vi "GHV232 CRAB.vi"() -> ()   [LabVIEW 2017]
doc: "The Basic Serial Read and Write example performs a Serial Port Read, a Serial Port Write, or a combination of these actions. The user selects the actions (read or write) on the front panel. If both are selected, the VI will write the data first, read data, and then close the VISA session that is opened to the port. This VI will wait until the specified number of bytes is received at the port. Only the number of bytes specified will be read.\n\nINSTRUCTIONS:\n1) Select the serial resource and configuration parameters (baud rate, data bits, parity, stop bits, flow control).\n2) Select the operations to be performed. \n3) Connect the serial port to your device. If no device is available, perform a loopback test by doing one of the following. Short pins 2 and 3 on a RS-232 cable or short pin 4 to pin 8 and pin 5 to pin 9 on a RS-485/422 cable. \n4) Run the VI to see the data read. (The \"read string\" will match the \"string to write\" if a loopback test was performed.)\n\nNote: The parameters set for the serial port must match the parameters of the connected instrument or device. In this example, the bytes to read parameter specifies the number of bytes that the serial port reads. If there were more bytes at the port than the number specified in bytes to read, those bytes would not be read. Also, if you specify to read more bytes than the number of bytes actually read, you might receive a timeout error message.\n\nOn the block diagram, the Configure Serial Port VI sets the configuration parameters. The front panel displays the controls used to configure the basic parameters, such as baud rate, data bits, and parity. Constants configure the other parameters the user probably does not need set. After the VISA Configure Serial Port VI opens the VISA session and configures the port, the VI passes the VISA resource name to other VIs that perform operations on that VISA resource. The VISA Write function sends a command to the serial device and the VISA Read function returns data based on the command. The VISA Close function then closes the reference to the serial device. It is important to close the reference; otherwise communication through with that port through protocols other than VISA might not be possible."
uses:
  <vilib>/Instr/_visa.llb/VISA Configure Serial Port (Instr).vi
  <vilib>/Analysis/1siggen.llb/Ramp Pattern by Delta.vi
  <vilib>/Analysis/NI_AALBase.lvlib
panel:
  in  "Send 3":bool
  out "Message 3":string
  in  "Reset 3":bool
  out "HV On 3":bool
  out "Fault 3":bool
  out "Vmode 3":bool
  out "Imode 3":bool
  out "Voltage Monitor 3":dbl format="%#.2g"
  out "Current Monitor 3":dbl format="%#.2g"
  in  "High Voltage 3":bool
  in  "Voltage Progra3":dbl min=0.0 max=100.0 step=0.1 format="%#.2g"
  in  "Current Progra3":dbl min=0.0 max=100.0 step=0.1 format="%#.2g"
  in  "Version 3":bool
  in  "?":bool
  in  "Baud Rate 3":u16=9600 min=1200 max=19200 step=1200
  in  "Flow Control 3":u16(ring) items=["None"=0, "XON/XOFF"=1, "RTS/CTS"=2, "DTR/DSR"=4]
  in  "Stop Bits 3":u16(ring)=10 items=["1.0"=10, "1.5"=15, "2.0"=20]
  in  "Parity 3":u16(ring) items=["None", "Odd", "Even", "Mark", "Space"]
  in  "Data Bits 3":u16=8 min=5 max=8 step=1
  in  "VISA resource name 3":refnum<visa-resource-name>="COM1"
  in  "Send 2":bool
  out "Message 2":string
  in  "Reset 2":bool
  out "HV On 2":bool
  out "Fault 2":bool
  out "Vmode 2":bool
  out "Imode 2":bool
  out "Voltage Monitor 2":dbl format="%#.2g"
  out "Current Monitor 2":dbl format="%#.2g"
  in  "High Voltage 2":bool
  in  "Voltage Program 2":dbl min=0.0 max=100.0 step=0.1 format="%#.2g"
  in  "Current Program 2":dbl min=0.0 max=100.0 step=0.1 format="%#.2g"
  in  "Version 2":bool
  in  "?":bool
  in  "Baud Rate 2":u16=9600 min=1200 max=19200 step=1200
  in  "Flow Control 2":u16(ring) items=["None"=0, "XON/XOFF"=1, "RTS/CTS"=2, "DTR/DSR"=4]
  in  "Stop Bits 2":u16(ring)=10 items=["1.0"=10, "1.5"=15, "2.0"=20]
  in  "Parity 2":u16(ring) items=["None", "Odd", "Even", "Mark", "Space"]
  in  "Data Bits 2":u16=8 min=5 max=8 step=1
  in  "VISA resource name 2":refnum<visa-resource-name>="COM1"
  in  "?":bool
  in  "Version":bool
  in  "Baud Rate":u16=9600 min=1200 max=19200 step=1200
  in  "Reset":bool
  in  "Send":bool
  in  "Flow Control":u16(ring) items=["None"=0, "XON/XOFF"=1, "RTS/CTS"=2, "DTR/DSR"=4]
  in  "Stop Bits":u16(ring)=10 items=["1.0"=10, "1.5"=15, "2.0"=20]
  in  "Parity":u16(ring) items=["None", "Odd", "Even", "Mark", "Space"]
  in  "Data Bits":u16=8 min=5 max=8 step=1
  in  "High Voltage":bool
  in  "Voltage Program":dbl min=0.0 max=100.0 step=0.1 format="%#.2g"
  in  "Current Program":dbl min=0.0 max=100.0 step=0.1 format="%#.2g"
  in  "VISA resource name":refnum<visa-resource-name>="COM1"
  out "Message":string
  out "Fault":bool
  out "HV On":bool
  out "Imode":bool
  out "Vmode":bool
  out "Current Monitor":dbl format="%#.2g"
  out "Voltage Monitor":dbl format="%#.2g"
  # "GHV232 Example:  When this example is run, it will continuously query the power supply and update the the digital and\nanalog monitors (0-100%).  The Send Program button will send the the programs (0-100%) and the high voltage enable\nsignal to the power supply.  A Power Supply Reset will set both voltage and current programs to zero and turn the high \nvoltage off.  The power supply will respond with 'Acknowledge OK' for both a Send Program and Power Supply Reset.  A \nFirmware Version Request will display the current revision of the Power Supply Firmware.  Disconnect will close the serial \nport and stop execution.  HV On, Fault, V/I Mode LEDs may not be available on all Power Supplies."
  # "GHV PowerSupply 6 EL+"
  # "GHV PowerSupply 5 FIELDCAGE"
  # "GHV PowerSupply 4 EL++"
  # "Programs"
  # "Programs"
  # "Programs"
  # "Configuration"
  # "Configuration"
  # "Configuration"
  # "%"
  # "On"
  # "On"
  # "On"
  # "%"
  # "%"
  # "%"
  # "Off"
  # "Off"
  # "Off"
  # "%"
  # "%"
  # "%"
  # "Monitors"
  # "Monitors"
  # "Monitors"
  # "%"
  # "%"
  # "%"
  # "%"
  # "%"
  # "%"
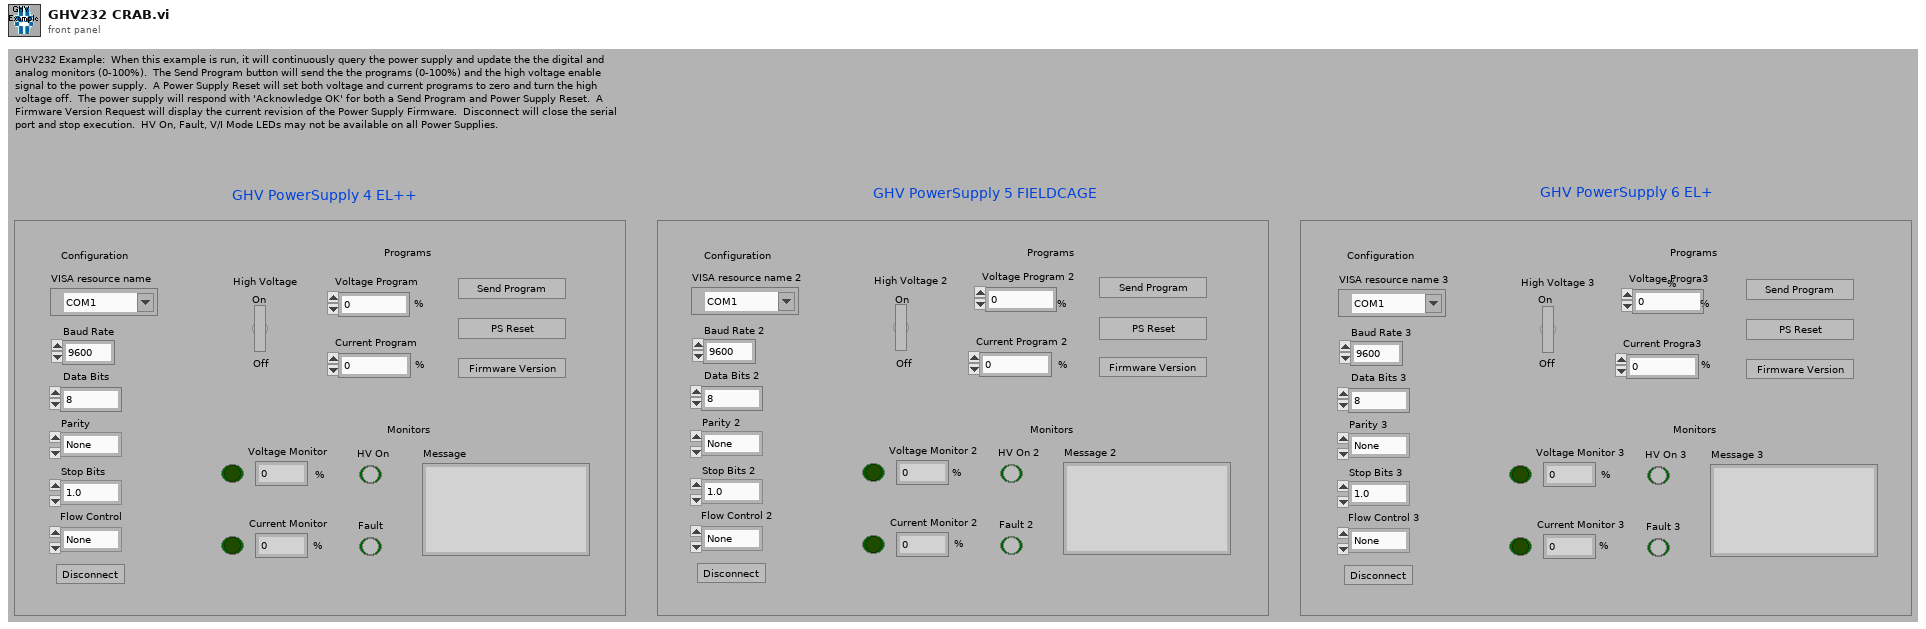
[diagram p1: front panel]
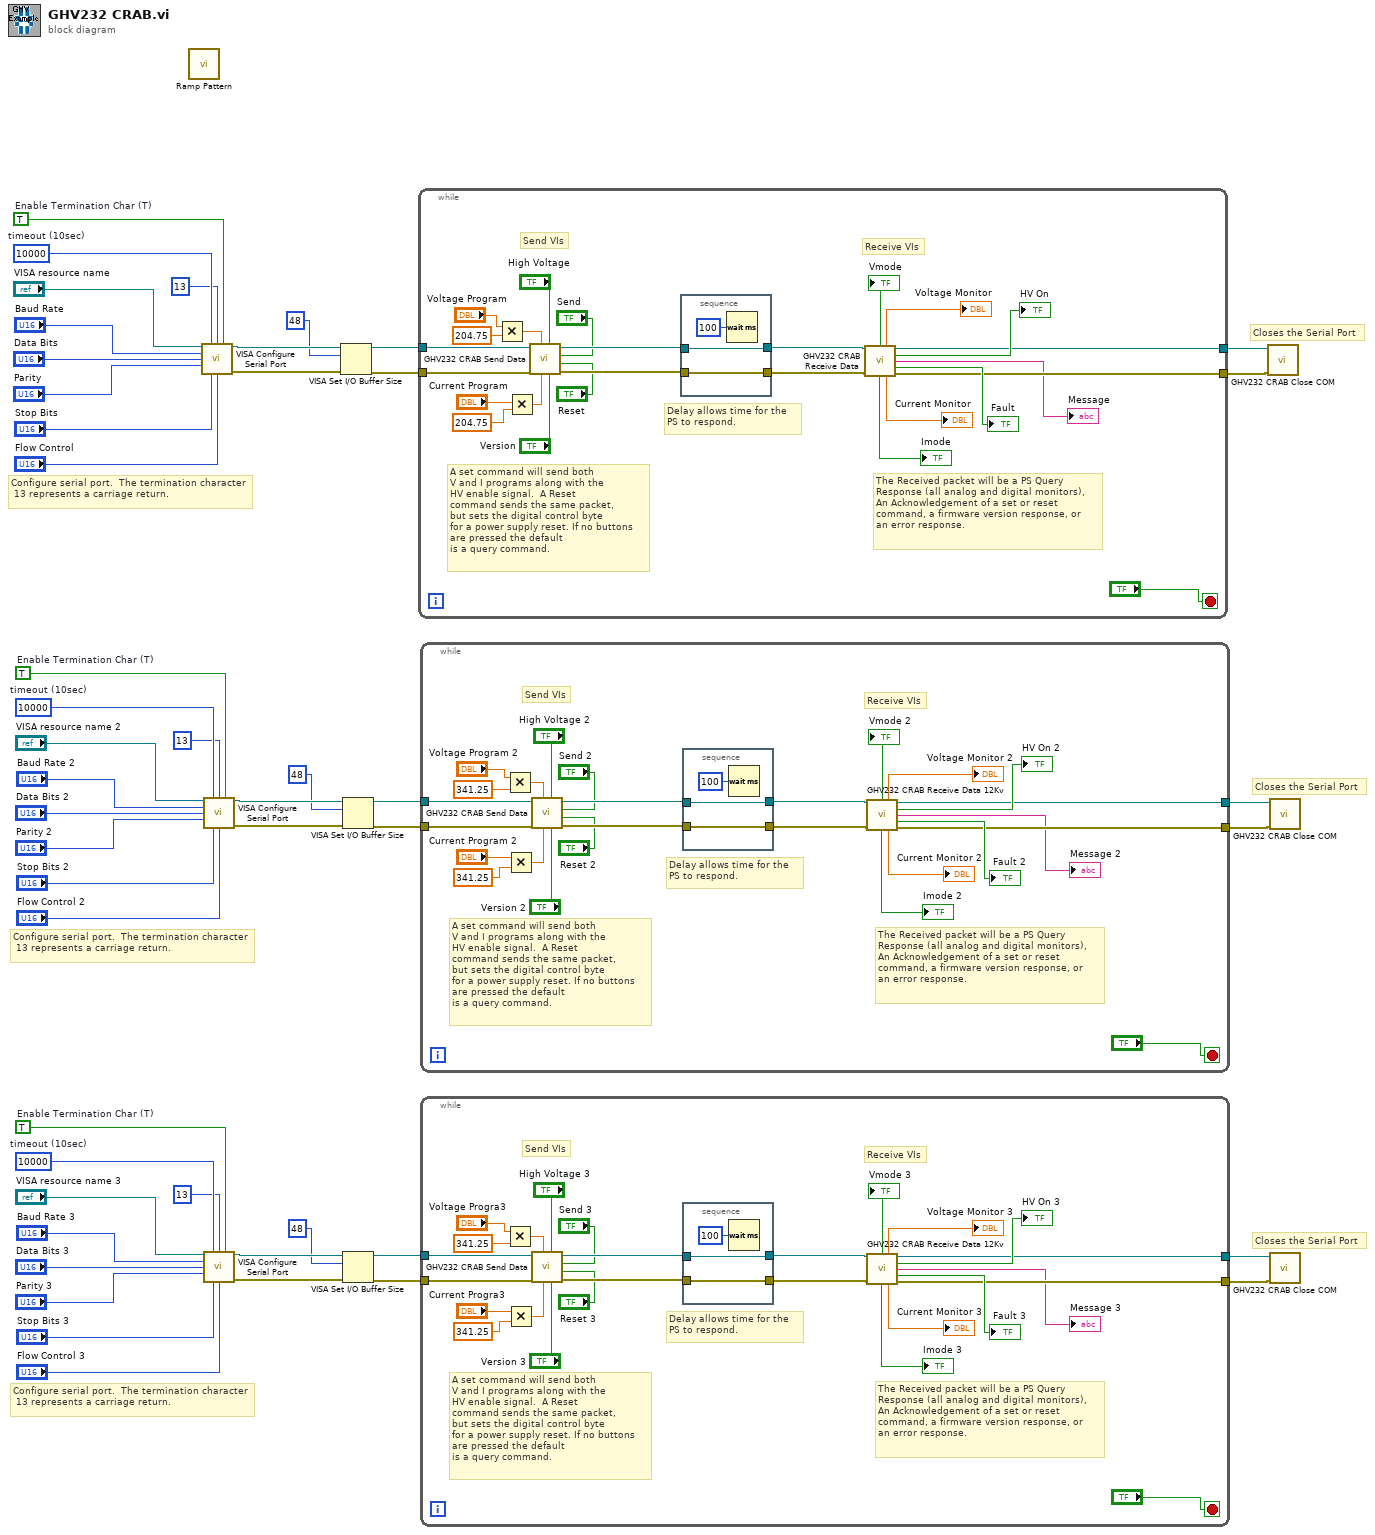
[diagram p0: block diagram]
diagram:
  w13 = TRUE  # Enable Termination Char (T)
  w14 = u32 10000  # timeout (10sec)
  w29 = TRUE  # Enable Termination Char (T)
  w30 = u32 10000  # timeout (10sec)
  w45 = TRUE  # Enable Termination Char (T)
  w46 = u32 10000  # timeout (10sec)
  # "Closes the Serial Port"
  # "Configure serial port.  The termination character\n 13 represents a carriage return."
  # "Closes the Serial Port"
  # "Configure serial port.  The termination character\n 13 represents a carriage return."
  # "Closes the Serial Port"
  # "Configure serial port.  The termination character\n 13 represents a carriage return."
  n1 = call-poly <vilib>:"Ramp Pattern.vi"() -> ()  [unwired: 9 in, 3 out]
  n2 = call-poly "VISA Configure Serial Port"("VISA resource name"="VISA resource name", "timeout (10sec)"=w46, "termination char\n(0xA = '\\n' = LF)"=13, "Enable Termination\nChar (T)"=w45, "baud rate (9600)"="Baud Rate", "data bits (8)"="Data Bits", "parity (0:none)"="Parity", "stop bits (10: 1 bit)"="Stop Bits", "flow control (0:none)"="Flow Control") -> ("VISA resource name out"=w35:refnum<visa-resource-name>, "error out"=w34:errorcluster)  [unwired: 5 in]
  n3 = call-poly "VISA Configure Serial Port"("VISA resource name"="VISA resource name 2", "timeout (10sec)"=w30, "termination char\n(0xA = '\\n' = LF)"=13, "Enable Termination\nChar (T)"=w29, "baud rate (9600)"="Baud Rate 2", "data bits (8)"="Data Bits 2", "parity (0:none)"="Parity 2", "stop bits (10: 1 bit)"="Stop Bits 2", "flow control (0:none)"="Flow Control 2") -> ("VISA resource name out"=w19:refnum<visa-resource-name>, "error out"=w18:errorcluster)  [unwired: 5 in]
  n4 = call-poly "VISA Configure Serial Port"("VISA resource name"="VISA resource name 3", "timeout (10sec)"=w14, "termination char\n(0xA = '\\n' = LF)"=13, "Enable Termination\nChar (T)"=w13, "baud rate (9600)"="Baud Rate 3", "data bits (8)"="Data Bits 3", "parity (0:none)"="Parity 3", "stop bits (10: 1 bit)"="Stop Bits 3", "flow control (0:none)"="Flow Control 3") -> ("VISA resource name out"=w3:refnum<visa-resource-name>, "error out"=w2:errorcluster)  [unwired: 5 in]
  n5 = VISA Set I/O Buffer Size(VISA resource name=w35, mask (16)=48, error in (no error)=w34) -> (VISA resource name out=w36:refnum<visa-resource-name>, error out=w37:errorcluster)  [unwired: 1 in]
  n6 = VISA Set I/O Buffer Size(VISA resource name=w19, mask (16)=48, error in (no error)=w18) -> (VISA resource name out=w20:refnum<visa-resource-name>, error out=w21:errorcluster)  [unwired: 1 in]
  n7 = VISA Set I/O Buffer Size(VISA resource name=w3, mask (16)=48, error in (no error)=w2) -> (VISA resource name out=w4:refnum<visa-resource-name>, error out=w5:errorcluster)  [unwired: 1 in]
  n8 = while {
    tunnel: w37 -> [w72]
    tunnel: w36 -> [w71]
    tunnel: [w62] -> w39
    tunnel: [w58] -> w38
    stop <- "?" stop-if-true
    # "The Received packet will be a PS Query\nResponse (all analog and digital monitors),\nAn Acknowledgement of a set or reset\ncommand, a firmware version response, or\nan error response."
    # "Delay allows time for the \nPS to respond."
    # "A set command will send both\nV and I programs along with the\nHV enable signal.  A Reset \ncommand sends the same packet,\nbut sets the digital control byte\nfor a power supply reset. If no buttons are pressed the default\nis a query command."
    # "Receive VIs"
    # "Send VIs"
    n9 = Multiply(x="Voltage Program", y=204.75) -> (x*y=w55:dbl)
    n10 = Multiply(x="Current Program", y=204.75) -> (x*y=w52:dbl)
    n11 = call "GHV232 CRAB Send Data.vi"("Reset"="Reset", "Send"="Send", "Version"="Version", "HV Enable"="High Voltage", "Current Program"=w52, "Voltage Program"=w55, "error in (no error)"=w72, "VISA resource name"=w71) -> ("error out"=w74:errorcluster, "VISA resource name 2"=w73:refnum<visa-resource-name>)  [unwired: 2 in]
    n12 = stacked-sequence {
      tunnel: [w77] -> w66
      tunnel: w73 -> [w77]
      tunnel: w74 -> [w76]
      tunnel: [w76] -> w65
      frame #0 {
        n13 = Wait (ms)(milliseconds to wait=100) -> ()  [unwired: 1 out]
      }
    }
    n14 = call "GHV232 CRAB Receive Data.vi"("VISA resource name"=w66, "error in (no error)"=w65) -> ("V"=→"Vmode":bool, "Vmon"=→"Voltage Monitor":dbl, "VISA resource name 2"=w62:refnum<visa-resource-name>, "HV on"=→"HV On":bool, "Message"=→"Message":string, "Fault"=→"Fault":bool, "I"=→"Imode":bool, "Imon"=→"Current Monitor":dbl, "error out"=w58:errorcluster)  [unwired: 5 in]
  }
  n15 = while {
    tunnel: w21 -> [w101]
    tunnel: w20 -> [w100]
    tunnel: [w91] -> w23
    tunnel: [w87] -> w22
    stop <- "?" stop-if-true
    # "The Received packet will be a PS Query\nResponse (all analog and digital monitors),\nAn Acknowledgement of a set or reset\ncommand, a firmware version response, or\nan error response."
    # "Delay allows time for the \nPS to respond."
    # "A set command will send both\nV and I programs along with the\nHV enable signal.  A Reset \ncommand sends the same packet,\nbut sets the digital control byte\nfor a power supply reset. If no buttons are pressed the default\nis a query command."
    # "Receive VIs"
    # "Send VIs"
    n16 = Multiply(x="Voltage Program 2", y=341.25) -> (x*y=w84:dbl)
    n17 = Multiply(x="Current Program 2", y=341.25) -> (x*y=w81:dbl)
    n18 = call "GHV232 CRAB Send Data.vi"("Reset"="Reset 2", "Send"="Send 2", "Version"="Version 2", "HV Enable"="High Voltage 2", "Current Program"=w81, "Voltage Program"=w84, "error in (no error)"=w101, "VISA resource name"=w100) -> ("error out"=w103:errorcluster, "VISA resource name 2"=w102:refnum<visa-resource-name>)  [unwired: 2 in]
    n19 = stacked-sequence {
      tunnel: [w106] -> w95
      tunnel: w102 -> [w106]
      tunnel: w103 -> [w105]
      tunnel: [w105] -> w94
      frame #0 {
        n20 = Wait (ms)(milliseconds to wait=100) -> ()  [unwired: 1 out]
      }
    }
    n21 = call "GHV232 CRAB Receive Data 12Kv.vi"("VISA resource name"=w95, "error in (no error)"=w94) -> ("V"=→"Vmode 2":bool, "Vmon"=→"Voltage Monitor 2":dbl, "VISA resource name 2"=w91:refnum<visa-resource-name>, "HV on"=→"HV On 2":bool, "Message"=→"Message 2":string, "Fault"=→"Fault 2":bool, "I"=→"Imode 2":bool, "Imon"=→"Current Monitor 2":dbl, "error out"=w87:errorcluster)  [unwired: 5 in]
  }
  n22 = while {
    tunnel: w5 -> [w130]
    tunnel: w4 -> [w129]
    tunnel: [w120] -> w7
    tunnel: [w116] -> w6
    stop <- "?" stop-if-true
    # "The Received packet will be a PS Query\nResponse (all analog and digital monitors),\nAn Acknowledgement of a set or reset\ncommand, a firmware version response, or\nan error response."
    # "Delay allows time for the \nPS to respond."
    # "A set command will send both\nV and I programs along with the\nHV enable signal.  A Reset \ncommand sends the same packet,\nbut sets the digital control byte\nfor a power supply reset. If no buttons are pressed the default\nis a query command."
    # "Receive VIs"
    # "Send VIs"
    n23 = Multiply(x="Voltage Progra3", y=341.25) -> (x*y=w113:dbl)
    n24 = Multiply(x="Current Progra3", y=341.25) -> (x*y=w110:dbl)
    n25 = call "GHV232 CRAB Send Data.vi"("Reset"="Reset 3", "Send"="Send 3", "Version"="Version 3", "HV Enable"="High Voltage 3", "Current Program"=w110, "Voltage Program"=w113, "error in (no error)"=w130, "VISA resource name"=w129) -> ("error out"=w132:errorcluster, "VISA resource name 2"=w131:refnum<visa-resource-name>)  [unwired: 2 in]
    n26 = stacked-sequence {
      tunnel: [w135] -> w124
      tunnel: w131 -> [w135]
      tunnel: w132 -> [w134]
      tunnel: [w134] -> w123
      frame #0 {
        n27 = Wait (ms)(milliseconds to wait=100) -> ()  [unwired: 1 out]
      }
    }
    n28 = call "GHV232 CRAB Receive Data 12Kv.vi"("VISA resource name"=w124, "error in (no error)"=w123) -> ("V"=→"Vmode 3":bool, "Vmon"=→"Voltage Monitor 3":dbl, "VISA resource name 2"=w120:refnum<visa-resource-name>, "HV on"=→"HV On 3":bool, "Message"=→"Message 3":string, "Fault"=→"Fault 3":bool, "I"=→"Imode 3":bool, "Imon"=→"Current Monitor 3":dbl, "error out"=w116:errorcluster)  [unwired: 5 in]
  }
  n29 = call "GHV232 CRAB Close COM.vi"("error in (no error)"=w38, "VISA resource name"=w39) -> ()  [unwired: 9 in, 1 out]
  n30 = call "GHV232 CRAB Close COM.vi"("error in (no error)"=w22, "VISA resource name"=w23) -> ()  [unwired: 9 in, 1 out]
  n31 = call "GHV232 CRAB Close COM.vi"("error in (no error)"=w6, "VISA resource name"=w7) -> ()  [unwired: 9 in, 1 out]
